vi "Create table test.vi"() -> ()   [LabVIEW 2017]
uses:
  <vilib>/addons/database/NI_Database_API.lvlib
  <vilib>/addons/database/Auxilliary.llb/DB Tools DataTypes.ctl
  <vilib>/addons/database/Auxilliary.llb/DB Tools Column Info.ctl
  SQL/SQL_DB-Enum.ctl
  Detailed Report/Controls/Detailed_Reports_Columns.ctl
  Detailed Report _Colums_Informatin.ctl
panel:
  out "Array 2":T2(array[cluster])
  out "error in (no error) 2":errorcluster
  out "columns":string[](array[string])
  out "tables":string[](array[string])
  out "error out":errorcluster
  in  "error in (no error)":errorcluster
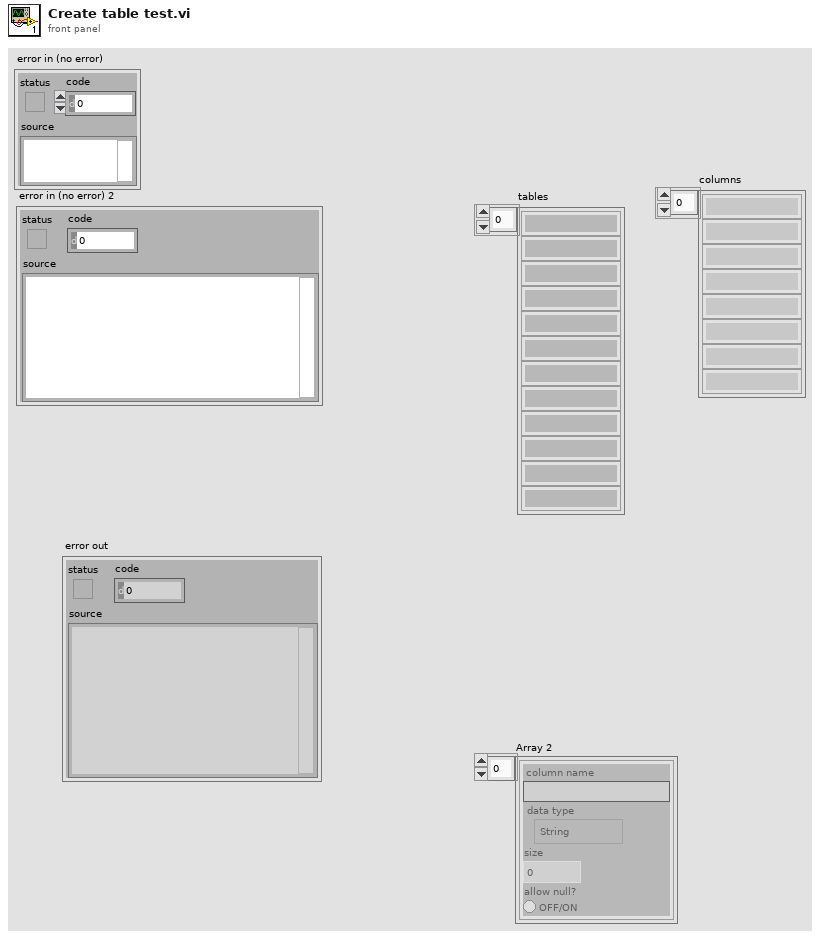
[diagram p1: front panel]
types:
  T1 = typedef "NI_Database_API.lvlib/DB Tools DataTypes.ctl" = enum16{"String", "Long (I32)", "Single (SGL)", "Double (DBL)", "Date/Time", "Binary"}
  T2 = cluster{"column name":string, "data type":T1, "size":i32, "allow null?":bool}[]
  T3 = typedef "Detailed_Reports_Columns.ctl" = string[]
  T4 = typedef "SQL_DB-Enum.ctl" = enum16{"INI DATA", "Open Connections", "Query", "Update Table", "Get Full Report", "Get Serial Numbers", "Get Table Columns", "Get Table Names", "Check & Create Table", "Close Connection"}
  T5 = typedef "Detailed Report _Colums_Informatin.ctl" = cluster{"column name":string, "data type":T1, "size":i32, "allow null?":bool}[]
  T6 = typedef "NI_Database_API.lvlib/DB Tools Column Info.ctl" = cluster{"column name":string, "data type":T1, "size":i32, "allow null?":bool}
  T7 = typedef "NI_Database_API.lvlib/Conn ObjectReference.ctl" = refnum<k1>
  T8 = cluster{"column name":string, "data type":T1, "size":i32, "allow null?":bool}
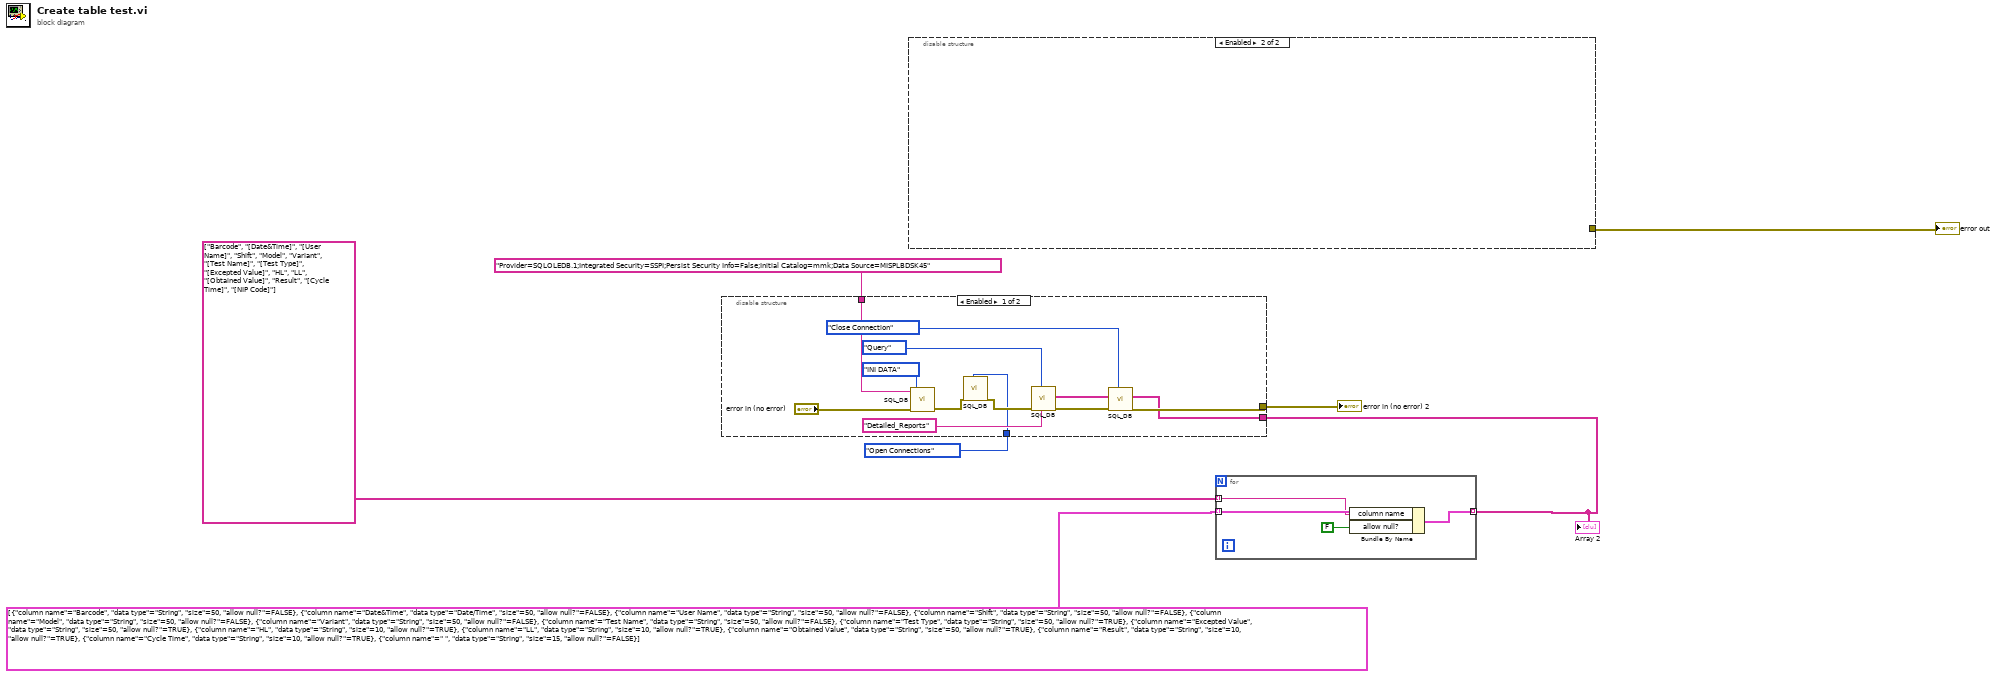
[diagram p0: block diagram]
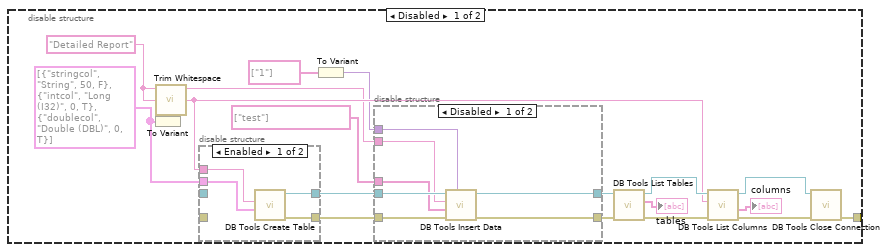
[diagram p2: hidden frame]
diagram:
  n1 = disable-structure shown="Enabled" {
    disable-tunnel: "Provider=SQLOLEDB.1;Integrated Security=SSPI;Persist Security Info=False;Initial Catalog=mmk;Data Source=MISPLBDSK45" -> [w17 _]
    disable-tunnel: [w12 _] -> w5
    disable-tunnel: [w11 _] -> w3
    disable-tunnel: SQL_DB-Enum."Open Connections" ("CTRL") -> [w8 _]
    frame Enabled {
      n2 = call "SQL_DB.vi"("CTRL"=SQL_DB-Enum."INI DATA", "error in (no error)"="error in (no error)", "Connection Info"=w17) -> ("error in (no error) 2"=w10:errorcluster)  [unwired: 6 in, 2 out]
      n3 = call "SQL_DB.vi"("CTRL"=w8, "error in (no error)"=w10) -> ("error in (no error) 2"=w9:errorcluster)  [unwired: 7 in, 2 out]
      n4 = call "SQL_DB.vi"("Table Name"="Detailed_Reports" ("table"), "CTRL"=SQL_DB-Enum."Query", "error in (no error)"=w9) -> ("error in (no error) 2"=w16:errorcluster, "Table/Columns"=w11:string[])  [unwired: 6 in, 1 out]
      n5 = call "SQL_DB.vi"("CTRL"=SQL_DB-Enum."Close Connection", "error in (no error)"=w16) -> ("error in (no error) 2"=w12:errorcluster)  [unwired: 7 in, 2 out]
    }
    frame Disabled {
    }
  }
  "error in (no error) 2" <- w5
  "Array 2" <- w3
  n6 = disable-structure shown="Enabled" {
    disable-tunnel: [w36 _] -> w7
    frame Disabled {
      w20 = "Detailed Report" ("table")
      w30 = T6[] [{"column name"="stringcol", "data type"=enum."String", "size"=50, "allow null?"=FALSE}, {"column name"="intcol", "data type"=enum."Long (I32)", "size"=0, "allow null?"=TRUE}, {"column name"="doublecol", "data type"=enum."Double (DBL)", "size"=0, "allow null?"=TRUE}] ("column information")
      n7 = To Variant(anything=w30) -> ()  [unwired: 1 out]
      n8 = call <vilib>:"Trim Whitespace.vi"("string"=w20) -> ("trimmed string"=w28:string)  [unwired: 1 in]
      n9 = disable-structure shown="Enabled" {
        disable-tunnel: _ -> [_ w51]
        disable-tunnel: _ -> [_ w50]
        disable-tunnel: [w49 w51] -> w32
        disable-tunnel: [w48 w50] -> w34
        disable-tunnel: w28 -> [w47 _]
        disable-tunnel: w30 -> [w46 _]
        frame Enabled {
          n10 = call <vilib>:"DB Tools Create Table.vi"("column information"=w46, "table"=w47) -> ("error out"=w48:errorcluster, "connection reference out"=w49:T7)  [unwired: 6 in]
        }
        frame Disabled {
        }
      }
      n11 = To Variant(anything=string[] ["1"]) -> (Variant=w21:variant)
      n12 = disable-structure shown="Disabled" {
        disable-tunnel: w34 -> [w43 w44]
        disable-tunnel: [w42 w44] -> w33
        disable-tunnel: w32 -> [w41 w45]
        disable-tunnel: [w40 w45] -> w31
        disable-tunnel: w20 -> [w39 _]
        disable-tunnel: string[] ["test"] -> [w38 _]
        disable-tunnel: w21 -> [w37 _]
        frame Disabled {
          n13 = call <vilib>:"DB Tools Insert Data.vi"("data"=w37, "error in (no error)"=w43, "columns"=w38, "table"=w39, "connection reference"=w41) -> ("error out"=w42:errorcluster, "connection reference out"=w40:T7)  [unwired: 5 in]
        }
        frame Enabled {
        }
      }
      n14 = call <vilib>:"DB Tools List Tables.vi"("error in (no error)"=w33, "connection reference"=w31) -> ("error out"=w27:errorcluster, "tables"=→"tables":string[], "connection reference out"=w29:T7)  [unwired: 3 in]
      n15 = call <vilib>:"DB Tools List Columns.vi"("error in (no error)"=w27, "table"=w28, "connection reference"=w29) -> ("error out"=w26:errorcluster, "columns"=→"columns":string[], "connection reference out"=w25:T7)  [unwired: 1 in, 1 out]
      n16 = call <vilib>:"DB Tools Close Connection.vi"("error in (no error)"=w26, "connection reference"=w25) -> ("error out"=w36:errorcluster)  [unwired: 5 in]
    }
    frame Enabled {
    }
  }
  "error out" <- w7
  n17 = for {
    tunnel: T5 [{"column name"="Barcode", "data type"=enum."String", "size"=50, "allow null?"=FALSE}, {"column name"="Date&Time", "data type"=enum."Date/Time", "size"=50, "allow null?"=FALSE}, {"column name"="User Name", "data type"=enum."String", "size"=50, "allow null?"=FALSE}, {"column name"="Shift", "data type"=enum."String", "size"=50, "allow null?"=FALSE}, {"column name"="Model", "data type"=enum."String", "size"=50, "allow null?"=FALSE}, {"column name"="Variant", "data type"=enum."String", "size"=50, "allow null?"=FALSE}, {"column name"="Test Name", "data type"=enum."String", "size"=50, "allow null?"=FALSE}, {"column name"="Test Type", "data type"=enum."String", "size"=50, "allow null?"=TRUE}, {"column name"="Excepted Value", "data type"=enum."String", "size"=50, "allow null?"=TRUE}, {"column name"="HL", "data type"=enum."String", "size"=10, "allow null?"=TRUE}, {"column name"="LL", "data type"=enum."String", "size"=10, "allow null?"=TRUE}, {"column name"="Obtained Value", "data type"=enum."String", "size"=50, "allow null?"=TRUE}, {"column name"="Result", "data type"=enum."String", "size"=10, "allow null?"=TRUE}, {"column name"="Cycle Time", "data type"=enum."String", "size"=10, "allow null?"=TRUE}, {"column name"=" ", "data type"=enum."String", "size"=15, "allow null?"=FALSE}] ("Array") -> [w55] mode=indexing
    tunnel: w3 -> [w54] mode=indexing
    tunnel: T3 ["Barcode", "[Date&Time]", "[User Name]", "Shift", "Model", "Variant", "[Test Name]", "[Test Type]", "[Excepted Value]", "HL", "LL", "[Obtained Value]", "Result", "[Cycle Time]", "[NIP Code]"] ("Column Names") -> [w52] mode=indexing
    n18 = Bundle By Name(cluster=w55, "column name"=w52, "allow null?"=FALSE) -> (w54:T8)
  }
